vi "gowave.vi"(1 "error in (no error)":errorcluster, 2 "Destination Wavelength":dbl format="%.4f") -> (0 "error out":errorcluster)   [LabVIEW 2017]
doc: "Positions the Monochromator to the Destination Wavelength \n\nDOES NOT RETUTRN UNTIL MONO IS IN POSITION, see slewtowave.vi for alternate.\nReturns No Eror in error out for success, See Error Codes\n(The global Wavelength Units determines units)"
uses:
  m_globals.vi
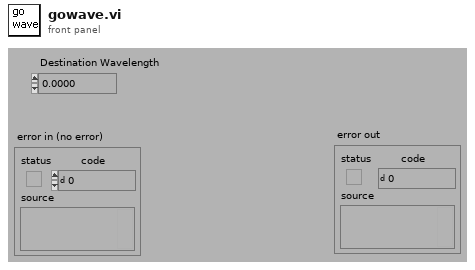
[diagram p1: front panel]
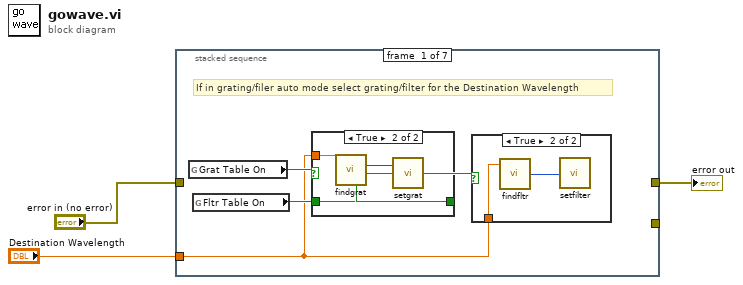
[diagram p0: block diagram]
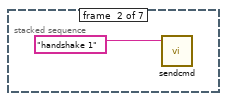
[diagram p4: hidden frame]
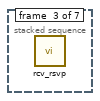
[diagram p5: hidden frame]
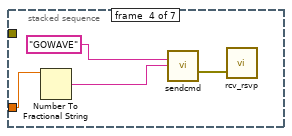
[diagram p6: hidden frame]
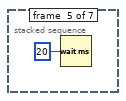
[diagram p7: hidden frame]
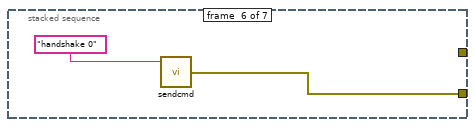
[diagram p8: hidden frame]
diagram:
  n1 = stacked-sequence {
    tunnel: "error in (no error)" -> [_ _ _ _ _ _ w22]
    tunnel: [_ _ _ _ _ _ w22] -> w2
    tunnel: "Destination Wavelength" -> [w4 _ _ w18 _ _ _]
    tunnel: [_ _ _ _ _ w20 _] -> _
    frame #0 {
      # "If in grating/filer auto mode select grating/filter for the Destination Wavelength"
      n2 = global read "m_globals.vi" "Grat Table On"() -> (w7:bool)
      n3 = global read "m_globals.vi" "Fltr Table On"() -> (w6:bool)
      n4 = case shown="True" w7 {
        tunnel: w6 -> [w10 w12]
        tunnel: [w10 w12] -> w5
        tunnel: w4 -> [_ w11]
        frame False {
        }
        frame True {
          n5 = call "findgrat.vi"("Present Wavelength"=w11) -> ("Grating"=w13:i32)
          n6 = call "setgrat.vi"("Grating"=w13) -> ()  [unwired: 2 in, 1 out]
        }
      }
      n7 = case shown="True" w5 {
        tunnel: w4 -> [_ w8]
        frame False {
        }
        frame True {
          n8 = call "findfltr.vi"("Present Wavelength"=w8) -> ("Filter"=w9:i32)
          n9 = call "setfilter.vi"("Filter"=w9) -> ()  [unwired: 2 in, 1 out]
        }
      }
    }
    frame #1 {
      n10 = call "sendcmd.vi"("command in"="handshake 1") -> ()  [unwired: 2 in, 1 out]
    }
    frame #2 {
      n11 = call "rcv_rsvp.vi"() -> ()  [unwired: 2 in, 2 out]
    }
    frame #3 {
      n12 = Number To Fractional String(number=w18) -> (F-format string=w16:string)  [unwired: 3 in]
      n13 = call "sendcmd.vi"("parameter"=w16, "command in"="GOWAVE") -> ("error out"=w15:errorcluster)  [unwired: 1 in]
      n14 = call "rcv_rsvp.vi"("error in (no error)"=w15) -> ()  [unwired: 1 in, 2 out]
    }
    frame #4 {
      n15 = Wait (ms)(milliseconds to wait=u32 20) -> ()  [unwired: 1 out]
    }
    frame #5 {
      n16 = call "sendcmd.vi"("command in"="handshake 0") -> ("error out"=w20:errorcluster)  [unwired: 2 in]
    }
    frame #6 {
    }
  }
  "error out" <- w2
